vi "v5.0 .vi"() -> ()   [LabVIEW 2018]
uses:
  <vilib>/DAQmx/read.llb/DAQmx Read (Analog 1D DBL NChan 1Samp).vi
  <extravilib>/ChannelInstances/High Speed Stream-c(a[.](c(dbl,dbl,dbl,dbl)),stamp,a[.](dbl),c(dbl,dbl,dbl,dbl,dbl,dbl,dbl))/_Read For Replicate.vi
  <extravilib>/ChannelInstances/High Speed Stream-c(a[.](c(dbl,dbl,dbl,dbl)),stamp,a[.](dbl),c(dbl,dbl,dbl,dbl,dbl,dbl,dbl))/Instantiate.vi
  <extravilib>/ChannelInstances/High Speed Stream-c(a[.](c(dbl,dbl,dbl,dbl)),stamp,a[.](dbl),c(dbl,dbl,dbl,dbl,dbl,dbl,dbl))/)Channel.vi
  <extravilib>/ChannelInstances/High Speed Stream-c(a[.](c(dbl,dbl,dbl,dbl)),stamp,a[.](dbl),c(dbl,dbl,dbl,dbl,dbl,dbl,dbl))/Abort Signal/Init Signal.vi
  <vilib>/Utility/file.llb/Write Delimited Spreadsheet (string).vi
  <vilib>/DAQmx/create/channels.llb/DAQmx Create Channel (AI-Temperature-Thermocouple).vi
  <vilib>/DAQmx/configure/timing.llb/DAQmx Timing (Sample Clock).vi
  <vilib>/DAQmx/miscellaneous.llb/DAQmx Fill In Error Info.vi
  <extravilib>/ChannelInstances/High Speed Stream-c(a[.](c(dbl,dbl,dbl,dbl)),stamp,a[.](dbl),c(dbl,dbl,dbl,dbl,dbl,dbl,dbl)).lvlib
  <resource>/objmgr/daqmx.rc
panel:
  in  "stop":bool
  in  "Array":T1(array[cluster])
  out "AFR Display":T2(array[cluster])
  in  "Species List":string[][](table)=[["Custom", "9999999999"], ["Methanol", "6.47"], ["Butanol", "11.2"], ["Diesel", "14.5"], ["Gasoline", "14.7"], ["Propane", "15.67"], ["Methane", "13.19"], ["Hydrogen", "34.3"], ["Ammonia", "6.0466"], ["Pentane", "15.32"], ["Butane", "14.98"], ["Hexane", "15.24"], ["Ethanol", "9"]]
  in  "Tab Control":enum32{"Live Data", "Set Data"}(tab)
  out "Flowrate Data":T3(array[cluster])
  out "Actual Sample Rate":dbl
  out "Export Timestamp":timestamp format="%<%H:%M:%S>T"
  out "Rig Temperatures":T4
  out "UI Timestamp":timestamp format="%<%X\n%x>T"
  out "DAQ Timestamp":timestamp format="%<%H:%M:%S>T"
  in  "file path (dialog if empty)":path
  out "Enum":T5(ring)
  in  "Start Recording?":bool
  in  "Stop Recording?":bool
  in  "Flowrate Control":dbl
  out "Status":T6(ring)
  in  "OK Button":bool
  in  "DAQ Properties":cluster{"Sample Rate [Hz]":dbl}={"Sample Rate [Hz]"=1.0} {"Sample Rate [Hz]" min=0.1 max=10000.0 step=0.1}
  # "Line Data"
  # "Rig Temperatures [ °C]"
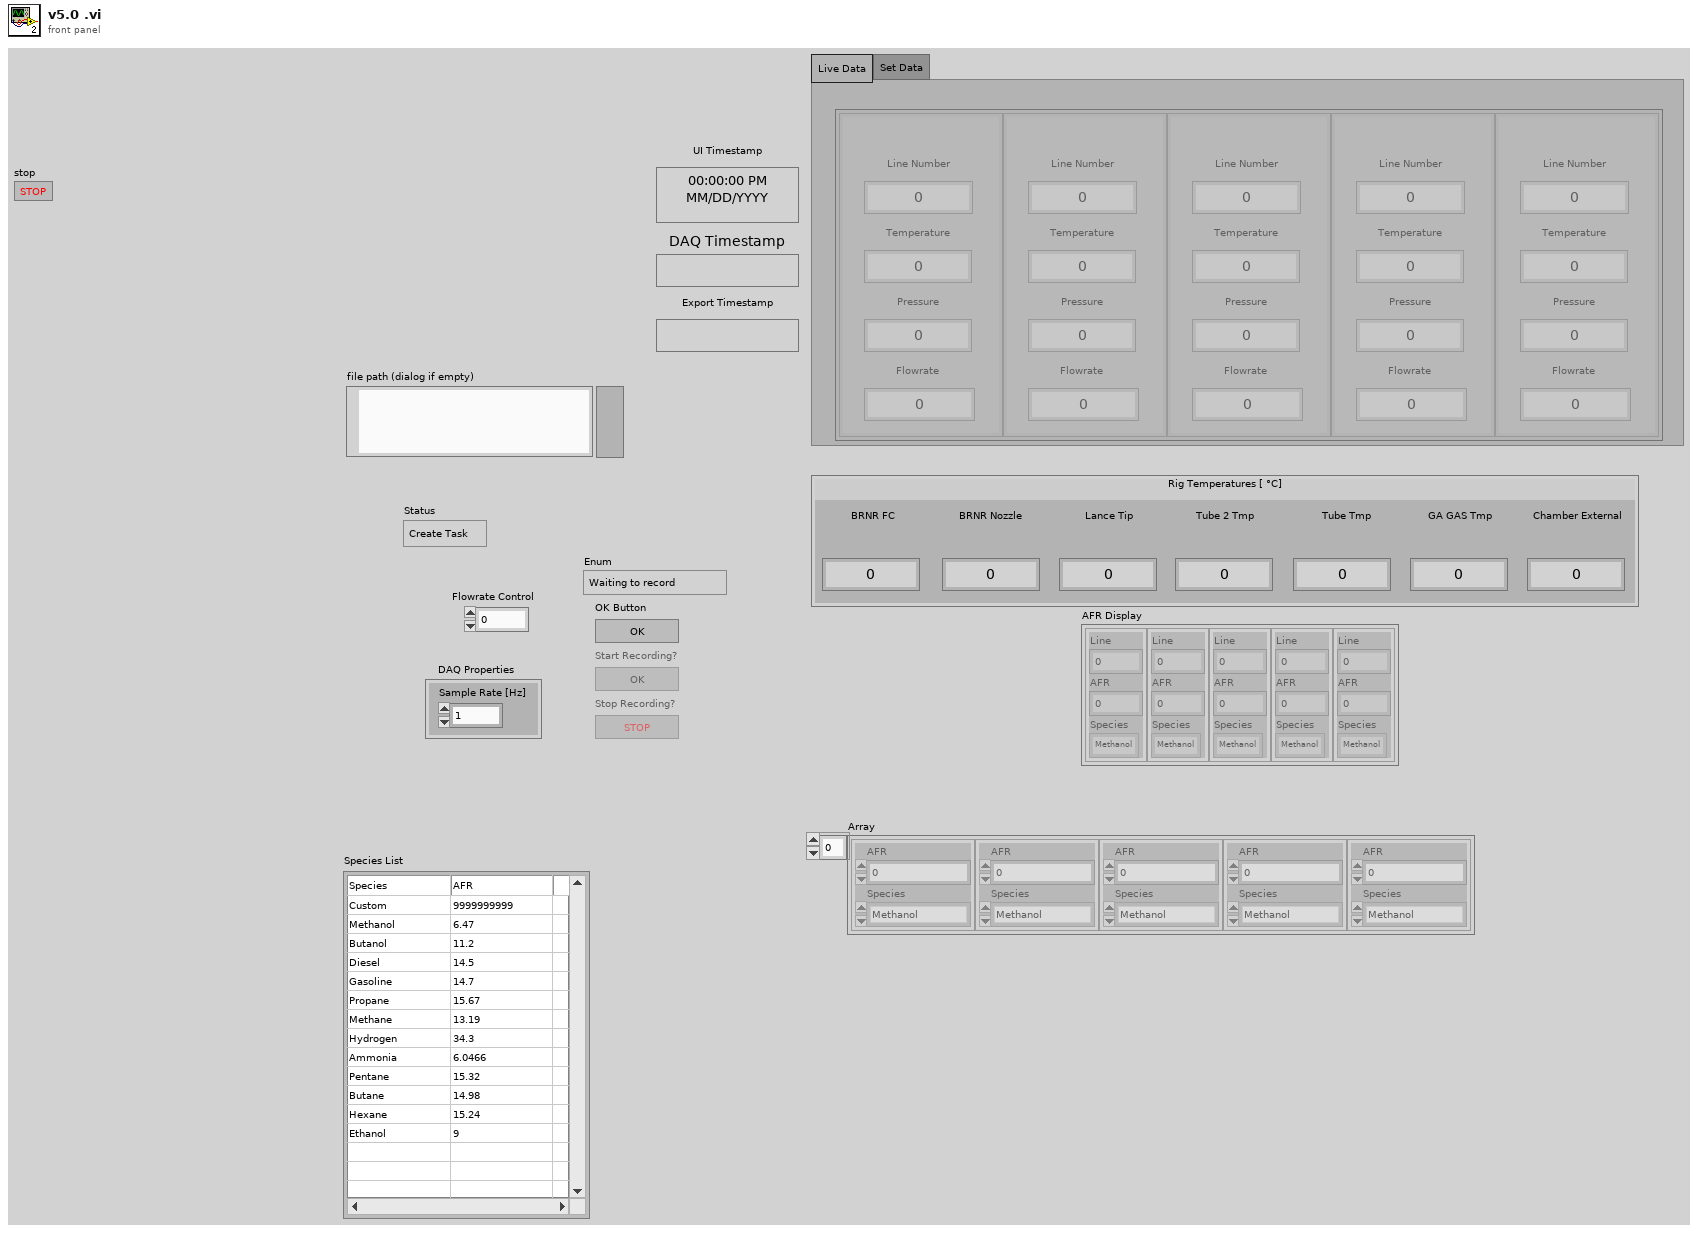
[diagram p1: front panel]
types:
  T1 = cluster{"AFR":dbl, "Species":enum16{"Methanol", "Ethanol", "Butanol", "Diesel", "Gasoline", "Propane", "Methane", "Hydrogen", "Pentane", "Butane", "Hexane", "Custom"}}[]
  T2 = cluster{"Line":i32, "AFR":dbl, "Species":enum16{"Methanol", "Ethanol", "Butanol", "Diesel", "Gasoline", "Propane", "Methane", "Hydrogen", "Pentane", "Butane", "Hexane", "Custom"}}[]
  T3 = cluster{"Line Number":dbl, "Temperature":dbl, "Pressure":dbl, "Flowrate":dbl}[]
  T4 = cluster{"BRNR FC":dbl, "BRNR Nozzle":dbl, "Lance Tip":dbl, "Tube 2 Tmp":dbl, "Tube Tmp":dbl, "GA GAS Tmp":dbl, "Chamber External":dbl}
  T5 = enum16{"Waiting to record", "Creating Spreadsheet", "Recording", "Finished Recording"}
  T6 = enum16{"Create Task", "Change Settings", "Check Settings", "Read Data", "End Task"}
  T7 = enum8{"Enabled", "Disabled", "Disabled and Grayed Out"}
  T8 = cluster{"Line":i32, "AFR":dbl, "Species":enum16{"Methanol", "Ethanol", "Butanol", "Diesel", "Gasoline", "Propane", "Methane", "Hydrogen", "Pentane", "Butane", "Hexane", "Custom"}}
  T9 = enum16{"Methanol", "Ethanol", "Butanol", "Diesel", "Gasoline", "Propane", "Methane", "Hydrogen", "Pentane", "Butane", "Hexane", "Custom"}
  T10 = cluster{"Flowrate Data":cluster{"Line Number":dbl, "Temperature":dbl, "Pressure":dbl, "Flowrate":dbl}[], "Current Time":timestamp, "DAQmx Data":dbl[], "Rig Temperatures":cluster{"BRNR FC":dbl, "BRNR Nozzle":dbl, "Lance Tip":dbl, "Tube 2 Tmp":dbl, "Tube Tmp":dbl, "GA GAS Tmp":dbl, "Chamber External Temp":dbl}}
  T11 = cluster{"BRNR FC":dbl, "BRNR Nozzle":dbl, "Lance Tip":dbl, "Tube 2 Tmp":dbl, "Tube Tmp":dbl, "GA GAS Tmp":dbl, "Chamber External Temp":dbl}
  T12 = typedef "High Speed Stream-c(a[.](c(dbl,dbl,dbl,dbl)),stamp,a[.](dbl),c(dbl,dbl,dbl,dbl,dbl,dbl,dbl)).lvlib/)Channel.ctl" = refnum<queue>
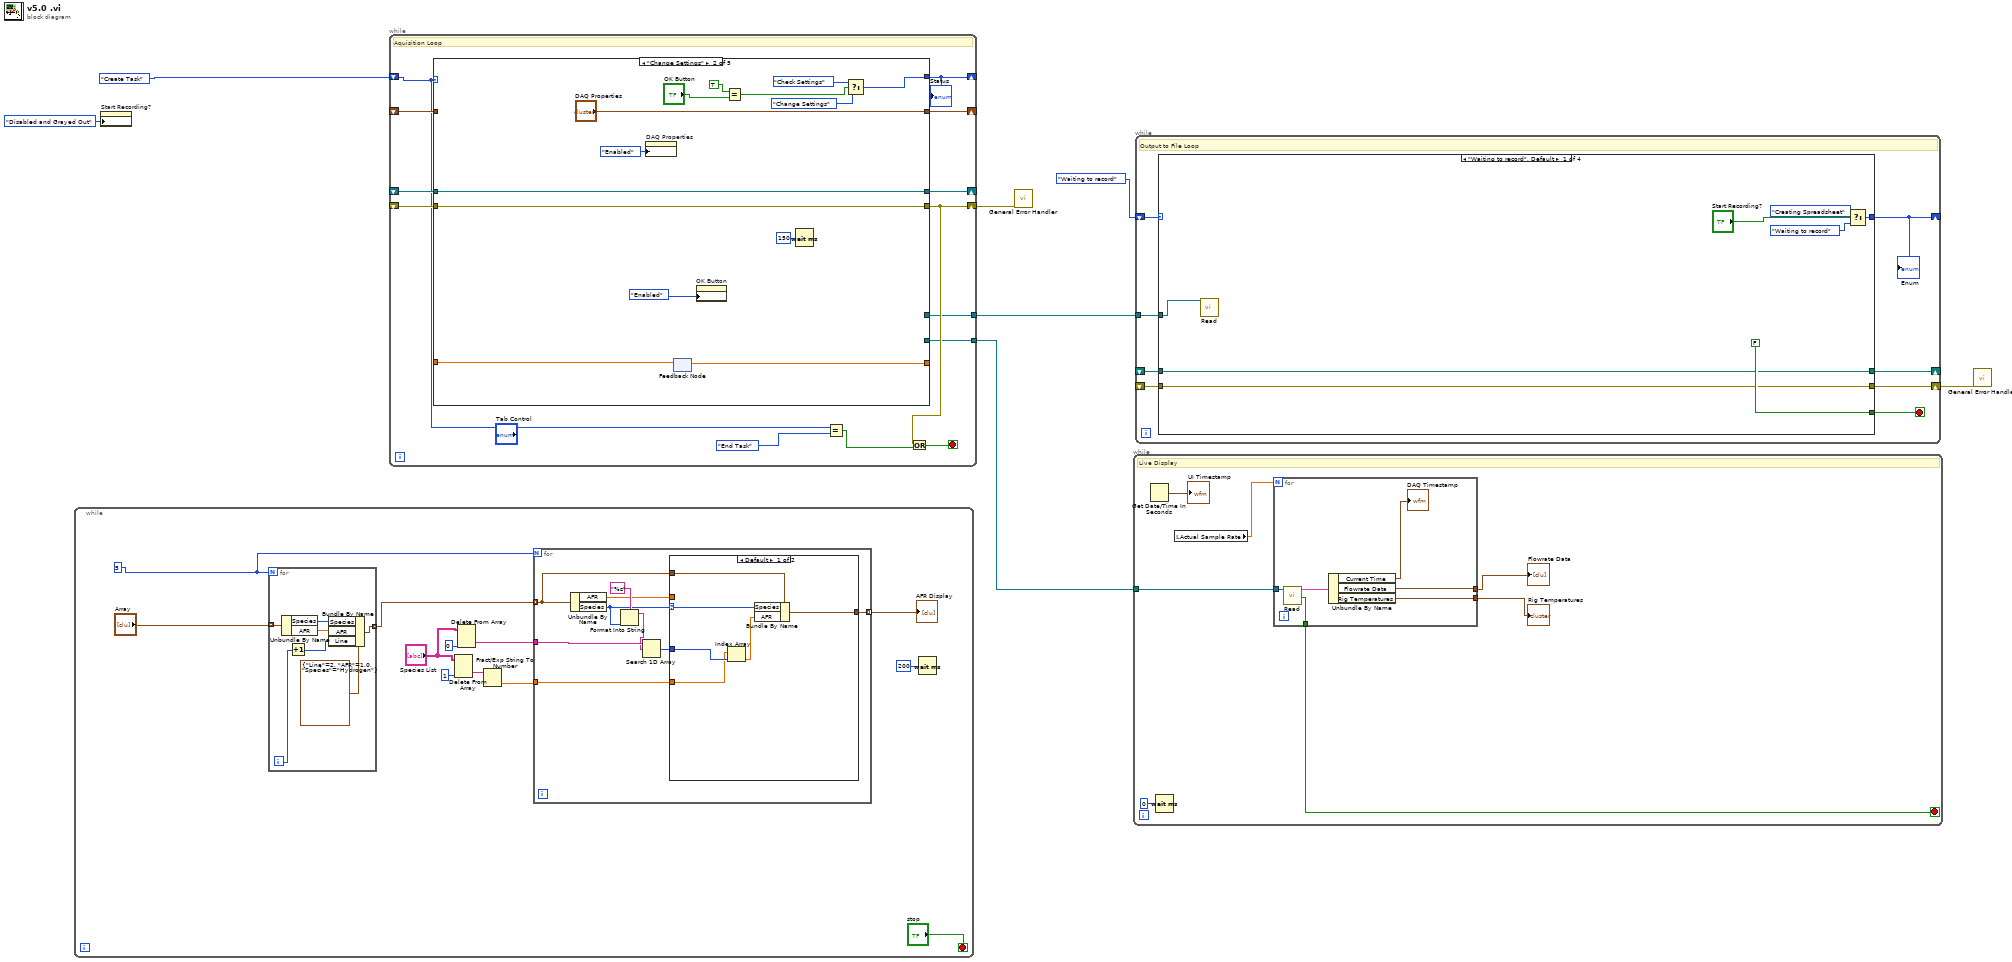
[diagram p0: block diagram]
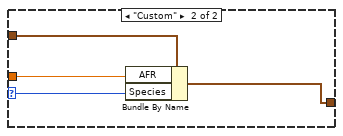
[diagram p2: hidden frame]
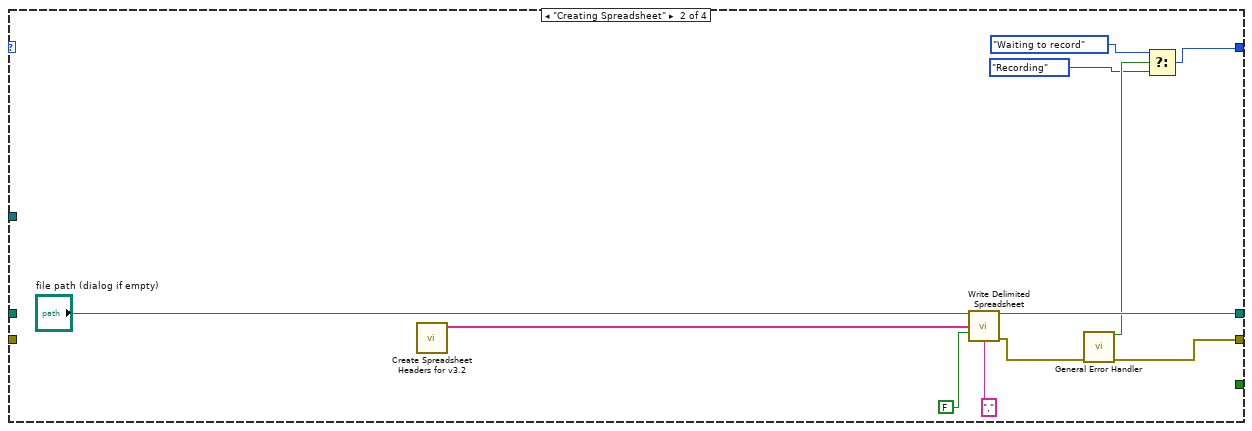
[diagram p3: hidden frame]
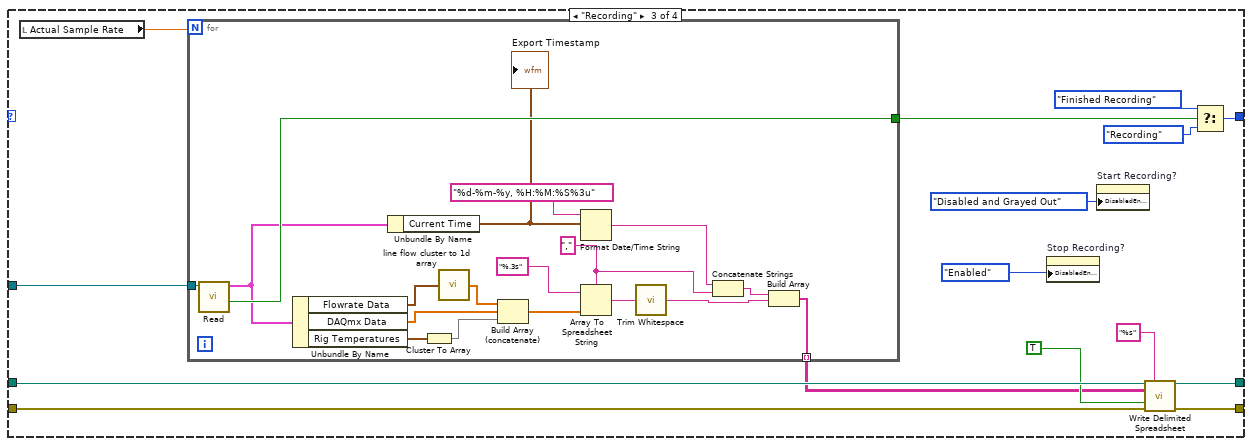
[diagram p4: hidden frame]
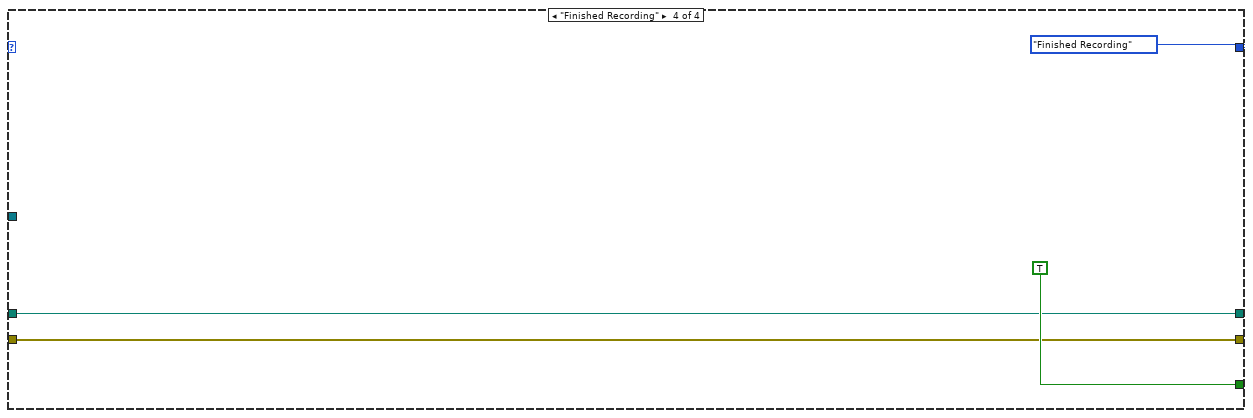
[diagram p5: hidden frame]
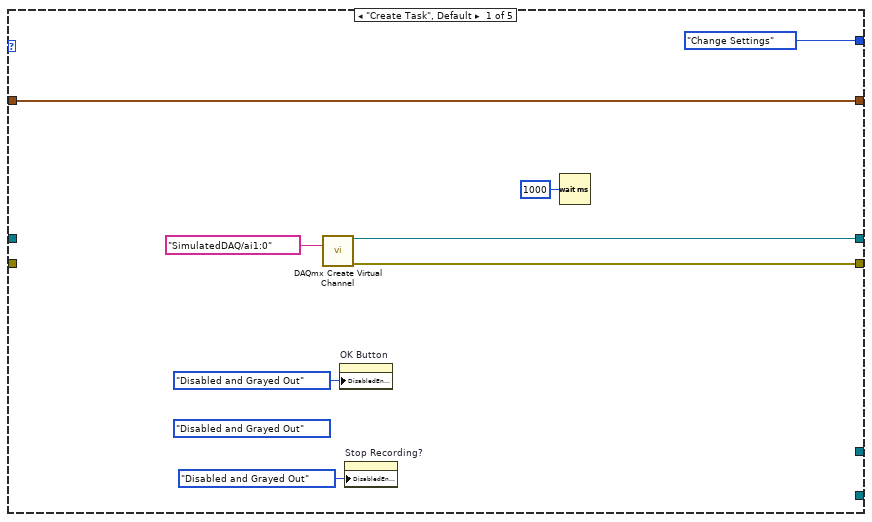
[diagram p6: hidden frame]
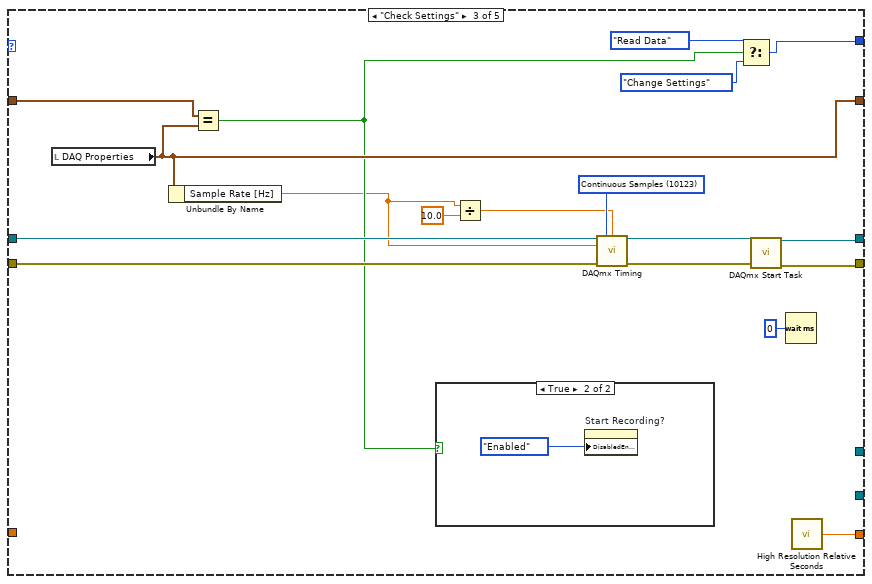
[diagram p7: hidden frame]
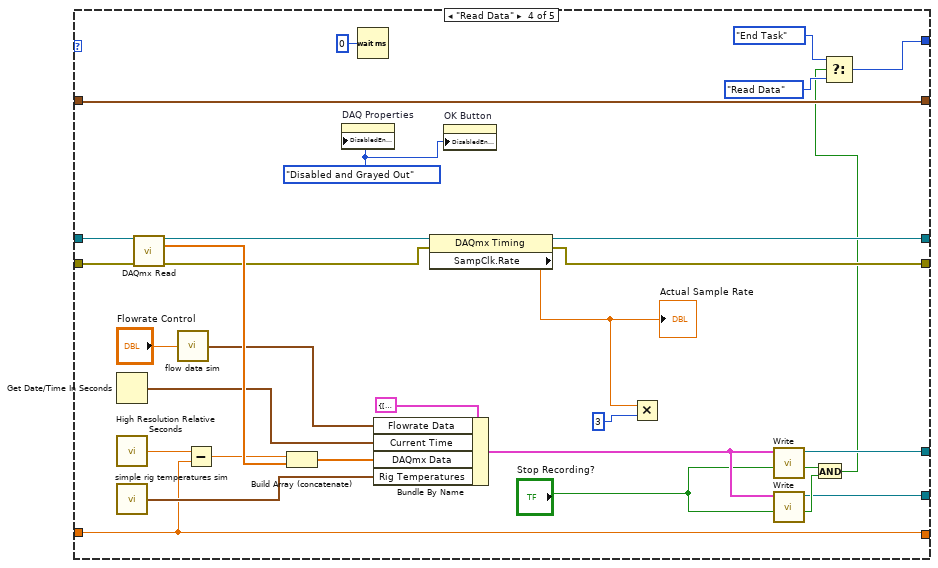
[diagram p9: hidden frame]
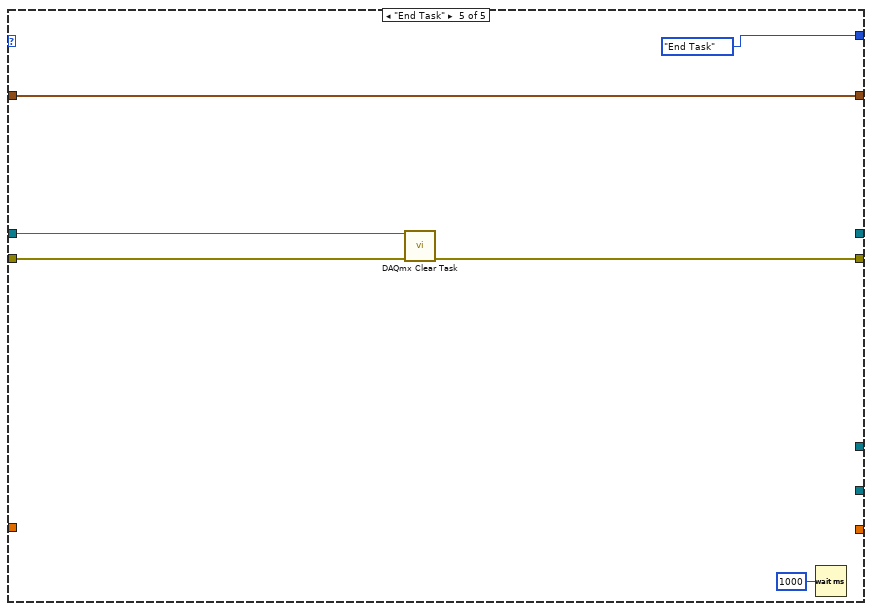
[diagram p10: hidden frame]
diagram:
  n1 = while {
    stop <- "stop" stop-if-true
    w10 = 5
    n2 = for {
      N: w10 -> [_]
      tunnel: "Array" -> [w26] mode=indexing
      tunnel: [w23] -> w11 mode=indexing
      i -> [w20]
      n3 = Unbundle By Name(w26) -> ("Species"=w25:T9, "AFR"=w24:dbl)
      n4 = Increment(x=w20) -> (x+1=w21:i32)
      n5 = Bundle By Name(cluster=T8 {"Line"=2, "AFR"=1.0, "Species"=enum."Hydrogen"} ("AFR Inputs"), "Species"=w25, "AFR"=w24, "Line"=w21) -> (w23:T8)
    }
    n6 = Delete From Array(array="Species List", index (col)=1 ("disabled index (col)")) -> (deleted portion=w14:string[])  [unwired: 2 in, 1 out]
    n7 = Delete From Array(array="Species List", index (col)=0) -> (deleted portion=w15:string[])  [unwired: 2 in, 1 out]
    n8 = Fract/Exp String To Number(string=w14) -> (number=w13:dbl[])  [unwired: 3 in, 1 out]
    n9 = for {
      N: w10 -> [_]
      tunnel: w15 -> [w34]
      tunnel: w13 -> [w31]
      tunnel: [w29] -> w9 mode=indexing
      tunnel: w11 -> [w28] mode=indexing
      n10 = Unbundle By Name(w28) -> ("AFR"=w32:dbl, "Species"=w27:T9)
      n11 = Format Into String(format string="%s", w27) -> (resulting string=w33:string)  [unwired: 2 in, 1 out]
      n12 = Search 1D Array(1D array=w34, element=w33) -> (index of element=w30:i32)  [unwired: 1 in]
      n13 = case shown="Default" w27 {
        selector: w27 -> [w41 w44]
        tunnel: w32 -> [_ w45]
        tunnel: w31 -> [w39 _]
        tunnel: w30 -> [w40 _]
        tunnel: [w37 w43] -> w29
        tunnel: w28 -> [w36 w42]
        frame Default {
          n14 = Index Array(array=w39, index=w40) -> (element=w38:dbl)
          n15 = Bundle By Name(cluster=w36, "Species"=w41, "AFR"=w38) -> (w37:T8)
        }
        frame "Custom" {
          n16 = Bundle By Name(cluster=w42, "AFR"=w45, "Species"=w44) -> (w43:T8)
        }
      }
    }
    "AFR Display" <- w9
    n17 = Wait (ms)(milliseconds to wait=u32 200) -> ()  [unwired: 1 out]
  }
  n18 = property on="Start Recording?" class="Bool"("DisabledEnum"=T7."Disabled and Grayed Out" ("Disabled")) -> ()  [unwired: 2 in, 2 out]
  n19 = while {
    shift-right: [w55] -> _
    shift-left: T6."Create Task" -> [w51]
    shift-right: [w60] -> _
    shift-left: _ -> [w58]
    shift-right: [w54] -> w3
    shift-left: _ -> [w57]
    shift-right: [w59] -> _
    shift-left: _ -> [w56]
    tunnel: [w50] -> w5
    tunnel: [w49] -> w1
    stop <- w46 stop-if-true
    # "Aquisition Loop"
    n20 = feedback #1() -> (w47:dbl)  [unwired: 1 in]
    n21 = case shown="\"Change Settings\"" w51 {
      tunnel: [w68 w80 w88 w110 _] -> w60
      tunnel: [w67 w79 w87 w111 w136] -> w54
      tunnel: [T6."Change Settings" w73 w94 w126 T6."End Task"] -> w55
      tunnel: [w64 "DAQ Properties" w91 w128 w135] -> w59
      tunnel: w58 -> [_ w80 w93 w130 w133]
      tunnel: w57 -> [_ w79 w92 w129 w132]
      tunnel: w56 -> [w64 _ w98 w128 w135]
      tunnel: [_ _ _ w117 _] -> w50
      tunnel: [_ _ _ w108 _] -> w49
      tunnel: [_ _ w81 w103 _] -> w48
      tunnel: w47 -> [_ _ _ w103 _]
      frame "Create Task", Default {
        (unwired) T7."Disabled and Grayed Out" ("Disabled")
        n22 = call-poly <vilib>:"DAQmx Create Virtual Channel.vi"("physical channels"=tag "SimulatedDAQ/ai1:0") -> ("task out"=w68:refnum<k21>, "error out"=w67:errorcluster)  [unwired: 13 in]
        n23 = property on="OK Button" class="Bool"("DisabledEnum"=T7."Disabled and Grayed Out" ("Disabled")) -> ()  [unwired: 2 in, 2 out]
        n24 = property on="Stop Recording?" class="Bool"("DisabledEnum"=T7."Disabled and Grayed Out" ("Disabled")) -> ()  [unwired: 2 in, 2 out]
        n25 = Wait (ms)(milliseconds to wait=u32 1000) -> ()  [unwired: 1 out]
      }
      frame "Change Settings" {
        n26 = property on="DAQ Properties" class="Clust (strict)"("DisabledEnum"=T7."Enabled" ("Disabled")) -> ()  [unwired: 2 in, 2 out]
        n27 = property on="OK Button" class="Bool"("DisabledEnum"=T7."Enabled" ("Disabled")) -> ()  [unwired: 2 in, 2 out]
        n28 = Equal?(x=TRUE, y="OK Button") -> (x = y?=w75:bool)
        n29 = Wait (ms)(milliseconds to wait=u32 150) -> ()  [unwired: 1 out]
        n30 = Select(t=T6."Check Settings", s=w75, f=T6."Change Settings") -> (s? t:f=w73:T6)
      }
      frame "Check Settings" {
        w86 = 10123 items=["Finite Samples"=10178, "Continuous Samples"=10123, "Hardware Timed Single Point"=12522] ("sample mode")
        n31 = local read "DAQ Properties"() -> (w91:cluster{"Sample Rate [Hz]":dbl})
        n32 = Unbundle By Name(w91) -> ("Sample Rate [Hz]"=w83:dbl)
        n33 = Equal?(x=w98, y=w91) -> (x = y?=w85:bool)
        n34 = case shown="True" w85 {
          frame False {
          }
          frame True {
            n35 = property on="Start Recording?" class="Bool"("DisabledEnum"=T7."Enabled" ("Disabled")) -> ()  [unwired: 2 in, 2 out]
          }
        }
        n36 = Divide(x=w83, y=10.0) -> (x/y=w82:dbl)
        n37 = call-poly <vilib>:"DAQmx Timing.vi"("task/channels in"=w93, "sample mode"=w86, "samples per channel"=w82, "rate"=w83, "error in"=w92) -> ("task out"=w90:refnum<k21>, "error out"=w89:errorcluster)  [unwired: 9 in]
        n38 = Select(t=T6."Read Data", s=w85, f=T6."Change Settings") -> (s? t:f=w94:T6)
        n39 = call <vilib>:"DAQmx Start Task.vi"("task/channels in"=w90, "error in"=w89) -> ("task out"=w88:refnum<k21>, "error out"=w87:errorcluster)  [unwired: 12 in]
        n40 = Wait (ms)(milliseconds to wait=u32 0) -> ()  [unwired: 1 out]
        n41 = call <vilib>:"High Resolution Relative Seconds.vi"() -> ("relative seconds"=w81:dbl)
      }
      frame "Read Data" {
        w116 = T7."Disabled and Grayed Out" ("Disabled")
        n42 = Get Date/Time In Seconds() -> (seconds since 1Jan1904=w120:timestamp)
        n43 = call <vilib>:"High Resolution Relative Seconds.vi"() -> ("relative seconds"=w107:dbl)
        n44 = call "simple rig temperatures sim.vi"() -> ("Rig Temperatures"=w118:T11)
        n45 = call-poly <vilib>:"DAQmx Read.vi"("task/channels in"=w130, "error in"=w129) -> ("task out"=w112:refnum<k21>, "data"=w123:dbl[], "error out"=w109:errorcluster)  [unwired: 11 in]
        n46 = call "flow data sim.vi"("Boondoggle Input"="Flowrate Control") -> ("Flowrate Data"=w119:T3)
        n47 = Subtract(x=w107, y=w103) -> (x-y=w104:dbl)
        n48 = Build Array (concatenate)(w104, w123) -> (w105:dbl[])
        n49 = property on="DAQ Properties" class="Clust (strict)"("DisabledEnum"=w116) -> ()  [unwired: 2 in, 2 out]
        n50 = Wait (ms)(milliseconds to wait=u32 0) -> ()  [unwired: 1 out]
        n51 = Bundle By Name(cluster=T10 {"Flowrate Data"=[{"Line Number"=1.0, "Temperature"=17.480721541683437, "Pressure"=24.0, "Flowrate"=0.0}, {"Line Number"=2.0, "Temperature"=21.850901927104296, "Pressure"=30.0, "Flowrate"=0.0}, {"Line Number"=3.0, "Temperature"=26.221082312525155, "Pressure"=36.0, "Flowrate"=0.0}, {"Line Number"=4.0, "Temperature"=30.591262697946018, "Pressure"=42.00000000000001, "Flowrate"=0.0}, {"Line Number"=5.0, "Temperature"=34.96144308336687, "Pressure"=48.0, "Flowrate"=0.0}], "Current Time"=timestamp(0 s since 1904-01-01), "DAQmx Data"=[], "Rig Temperatures"={"BRNR FC"=0.0, "BRNR Nozzle"=0.0, "Lance Tip"=0.0, "Tube 2 Tmp"=0.0, "Tube Tmp"=0.0, "GA GAS Tmp"=0.0, "Chamber External Temp"=0.0}}, "Flowrate Data"=w119, "Current Time"=w120, "DAQmx Data"=w105, "Rig Temperatures"=w118) -> (w115:T10)
        n52 = property class="DAQmx Timing"(reference=w112, error in=w109) -> (reference out=w110:refnum<k21>, error out=w111:errorcluster, "SampClk.Rate"=w102:dbl)
        "Actual Sample Rate" <- w102
        n53 = property on="OK Button" class="Bool"("DisabledEnum"=w116) -> ()  [unwired: 2 in, 2 out]
        n54 = Multiply(x=w102, y=3) -> ()  [unwired: 1 out]
        n55 = call <extravilib>:"Write.vi"("last element? (F)"="Stop Recording?", "element"=w115) -> ("done?"=w114:bool, "channel"=w117:T12)  [unwired: 7 in, 1 out]
        n56 = call <extravilib>:"Write.vi"("last element? (F)"="Stop Recording?", "element"=w115) -> ("done?"=w113:bool, "channel"=w108:T12)  [unwired: 7 in, 1 out]
        n57 = And(x=w114, y=w113) -> (x .and. y?=w106:bool)
        n58 = Select(t=T6."End Task", s=w106, f=T6."Read Data") -> (s? t:f=w126:T6)
      }
      frame "End Task" {
        n59 = call <vilib>:"DAQmx Clear Task.vi"("task in"=w133, "error in"=w132) -> ("error out"=w136:errorcluster)  [unwired: 13 in]
        n60 = Wait (ms)(milliseconds to wait=u32 1000) -> ()  [unwired: 1 out]
      }
    }
    "Status" <- w55
    n61 = feedback-in #1(w48) -> ()
    n62 = Equal?(x=w51, y=T6."End Task") -> (x = y?=w52:bool)
    n63 = Or(x=w54, y=w52) -> (x .or. y?=w46:bool)
  }
  n64 = call <vilib>:"General Error Handler.vi"("error in (no error)"=w3) -> ()  [unwired: 10 in, 5 out]
  n65 = while {
    tunnel: w1 -> [w140]
    stop <- w143 stop-if-true
    # "Live Display"
    n66 = Get Date/Time In Seconds() -> (seconds since 1Jan1904=→"UI Timestamp":timestamp)
    n67 = Wait (ms)(milliseconds to wait=u32 0) -> ()  [unwired: 1 out]
    n68 = local read "Actual Sample Rate"() -> (w139:dbl)
    n69 = for {
      N: w139 -> [_]
      tunnel: [w149] -> w143
      tunnel: w140 -> [w146]
      tunnel: [w145] -> w137
      tunnel: [w144] -> w138
      n70 = call <extravilib>:"Read.vi"("channel"=w146) -> ("done?"=w149:bool, "element"=w148:T10)  [unwired: 6 in, 3 out]
      n71 = Unbundle By Name(w148) -> ("Current Time"=→"DAQ Timestamp":timestamp, "Flowrate Data"=w145:T3, "Rig Temperatures"=w144:T11)
    }
    "Flowrate Data" <- w137
    "Rig Temperatures" <- w138
  }
  n72 = while {
    shift-right: [w157] -> _
    shift-left: T5."Waiting to record" -> [w156]
    tunnel: w5 -> [w154]
    shift-right: [w152] -> _
    shift-left: _ -> [w153]
    shift-right: [w151] -> w4
    shift-left: _ -> [w150]
    stop <- w155 stop-if-true
    # "Output to File Loop"
    n73 = case shown="\"Waiting to record\", Default" w156 {
      tunnel: [w162 w168 w190 T5."Finished Recording"] -> w157
      tunnel: [FALSE _ _ TRUE] -> w155
      tunnel: w154 -> [w158 _ w187 _]
      tunnel: w153 -> [w160 _ w184 w211]
      tunnel: [w160 w176 w185 w211] -> w152
      tunnel: [w159 w170 w180 w210] -> w151
      tunnel: w150 -> [w159 _ w183 w210]
      frame "Waiting to record", Default {
        n74 = call <extravilib>:"Read.vi"("channel"=w158) -> ()  [unwired: 6 in, 5 out]
        n75 = Select(t=T5."Creating Spreadsheet", s="Start Recording?", f=T5."Waiting to record") -> (s? t:f=w162:T5)
      }
      frame "Creating Spreadsheet" {
        n76 = call "Create Spreadsheet Headers for v3.2.vi"() -> ("Array"=w175:string[])  [unwired: 11 in]
        n77 = call-poly <vilib>:"Write Delimited Spreadsheet.vi"("file path (dialog if empty)"="file path (dialog if empty)", "1D data"=w175, "append to file? (new file:F)"=FALSE, "delimiter (\\t)"="," ("delimiter (\\t)")) -> ("new file path (Not A Path if cancelled)"=w176:path, "error out"=w171:errorcluster)  [unwired: 10 in]
        n78 = call <vilib>:"General Error Handler.vi"("error in (no error)"=w171) -> ("error?"=w169:bool, "error out"=w170:errorcluster)  [unwired: 10 in, 3 out]
        n79 = Select(t=T5."Waiting to record", s=w169, f=T5."Recording") -> (s? t:f=w168:T5)
      }
      frame "Recording" {
        n80 = local read "Actual Sample Rate"() -> (w177:dbl)
        n81 = for {
          N: w177 -> [_]
          tunnel: w187 -> [w208]
          tunnel: [w207] -> w186
          tunnel: [w192] -> w178 mode=indexing
          w197 = "," ("delimiter (Tab)")
          n82 = call <extravilib>:"Read.vi"("channel"=w208) -> ("done?"=w207:bool, "element"=w205:T10)  [unwired: 6 in, 3 out]
          n83 = Unbundle By Name(w205) -> ("Flowrate Data"=w206:T3, "DAQmx Data"=w203:dbl[], "Rig Temperatures"=w209:T11)
          n84 = Unbundle By Name(w205) -> ("Current Time"=w198:timestamp)
          "Export Timestamp" <- w198
          n85 = Cluster To Array(cluster=w209) -> (array=w204:dbl[])
          n86 = call "line flow cluster to 1d array.vi"("Flowrate Data"=w206) -> ("Array"=w202:dbl[])
          n87 = Build Array (concatenate)(w202, w203, w204) -> (w195:dbl[])
          n88 = Format Date/Time String(time format string (%c)="%d-%m-%y, %H:%M:%S%3u", seconds (now)=w198) -> (date/time string=w196:string)  [unwired: 1 in]
          n89 = Array To Spreadsheet String(delimiter (Tab)=w197, array=w195, 3:"%.3s" ("format string")) -> (spreadsheet string=w201:string)
          n90 = call <vilib>:"Trim Whitespace.vi"("string"=w201) -> ("trimmed string"=w193:string)  [unwired: 1 in]
          n91 = Concatenate Strings(w196, w197) -> (w194:string)
          n92 = Build Array(w194, w193) -> (w192:string[])
        }
        n93 = property on="Stop Recording?" class="Bool"("DisabledEnum"=T7."Enabled" ("Disabled")) -> ()  [unwired: 2 in, 2 out]
        n94 = property on="Start Recording?" class="Bool"("DisabledEnum"=T7."Disabled and Grayed Out" ("Disabled")) -> ()  [unwired: 2 in, 2 out]
        n95 = call-poly <vilib>:"Write Delimited Spreadsheet.vi"("file path (dialog if empty)"=w184, "format (%s)"="%s", "2D data"=w178, "append to file? (new file:F)"=TRUE, "error in (no error)"=w183) -> ("new file path (Not A Path if cancelled)"=w185:path, "error out"=w180:errorcluster)  [unwired: 9 in]
        n96 = Select(t=T5."Finished Recording", s=w186, f=T5."Recording") -> (s? t:f=w190:T5)
      }
      frame "Finished Recording" {
      }
    }
    "Enum" <- w157
  }
  n97 = call <vilib>:"General Error Handler.vi"("error in (no error)"=w4) -> ()  [unwired: 10 in, 5 out]
